vi "XY to Waveform (multiple).vi"(8 "error in (no error)":errorcluster, 11 "XY-data in":cluster{"X-array":dbl[], "Y-array":dbl[]}[](array[cluster]) {"Y-array" format="%.2p"; "X-array" format="%.2p"}) -> (0 "error out":errorcluster, 2 "Waveform cluster":cluster{"x0":dbl, "dx":dbl, "Y array":dbl[]}[](array[cluster]), 3 "Waveform out":waveform(dbl)[](array[waveform]))   [LabVIEW 2019, in "xy_utilities.lvlib"]
doc: "Convert array of <b>XY-data</b> to array of <b>Waveforms</b>"
uses:
  xy_utilities.lvlib
  Get X and Y.vi
  Get X and Y (single).vi
  Resample.vi
  Resample (single).vi
  Get X Array dx.vi
  <vilib>/measure/maresamp.llb/Resample Waveforms (single shot).vi
  <vilib>/measure/maresamp.llb/Resample Pair of Arrays (single shot).vi
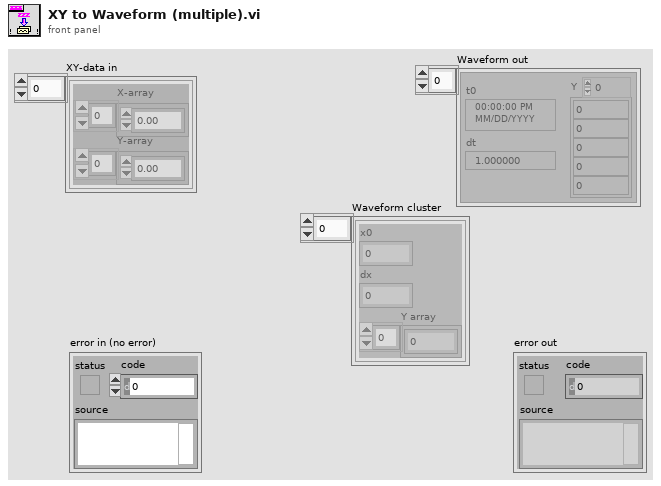
[diagram p1: front panel]
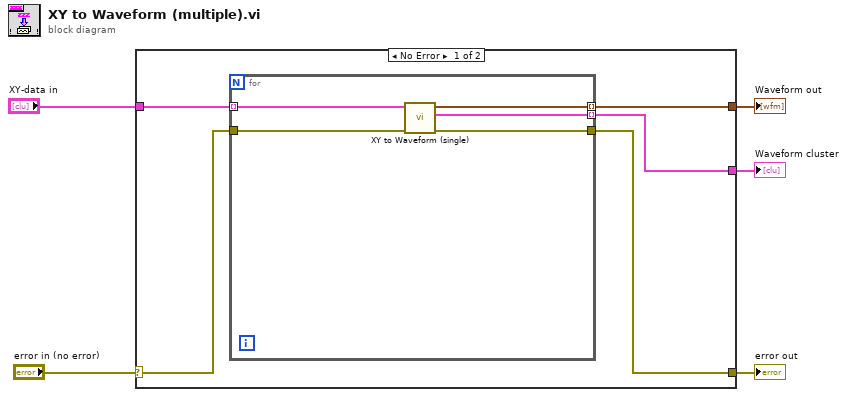
[diagram p0: block diagram]
diagram:
  n1 = case shown="No Error" "error in (no error)" {
    selector: "error in (no error)" -> [w6 w16]
    tunnel: [w7 w16] -> w4
    tunnel: "XY-data in" -> [w10 _]
    tunnel: [w8 _] -> w1
    tunnel: [w9 _] -> w2
    frame No Error {
      n2 = for {
        tunnel: w10 -> [w15] mode=indexing
        tunnel: [w14] -> w9 mode=indexing
        tunnel: [w13] -> w8 mode=indexing
        tunnel: w6 -> [w12]
        tunnel: [w11] -> w7
        n3 = call "XY to Waveform (single).vi"("error in (no error)"=w12, "XY-data in"=w15) -> ("error out"=w11:errorcluster, "Waveform cluster"=w13:cluster{"x0":dbl, "dx":dbl, "Y array":dbl[]}, "Waveform out"=w14:waveform(dbl))  [unwired: 7 in]
      }
    }
    frame Error {
    }
  }
  "error out" <- w4
  "Waveform out" <- w2
  "Waveform cluster" <- w1
